vi "Write Player Info.vi"(8 "error in (no error)":errorcluster, 10 "Player Info":T1={"Name"="Sleepy Engineer", "Color Box"=6618880, "Gloat Phrase"="All your base are belong to us!!"}, 11 "Mother in":refnum<class "Mother.lvclass">) -> (0 "error out":errorcluster, 3 "Mother out":refnum<class "Mother.lvclass">)   [LabVIEW 2014, in "Mother.lvclass"]
uses:
  Mother.lvclass
  Player Info.ctl
  Runner.lvclass
  SquareBattle.lvclass
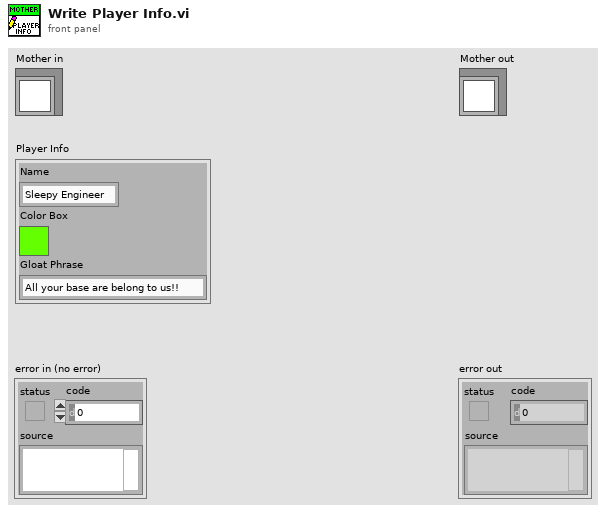
[diagram p1: front panel]
types:
  T1 = typedef "SquareBattle.lvclass/Player Info.ctl" = cluster{"Name":string, "Color Box":u32, "Gloat Phrase":string}
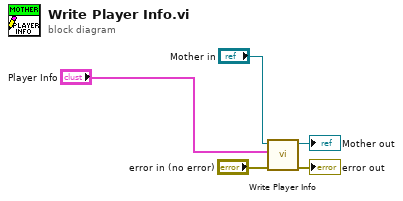
[diagram p0: block diagram]
diagram:
  n1 = call-parent "Write Player Info.vi"("error in (no error)"="error in (no error)", "Player Info"="Player Info", "Runner in"="Mother in") -> ("error out"=→"error out":errorcluster, "Runner out"=→"Mother out":refnum<class "Mother.lvclass">)  [unwired: 7 in]
